vi "Do.vi"(8 "error in (no error)":errorcluster, 10 "Actor in":refnum<class "Actor.lvclass">, 11 "Measure Msg":refnum<class "Measure Msg.lvclass">) -> (0 "error out":errorcluster, 2 "Actor out":refnum<class "Actor.lvclass">)   [LabVIEW 2015, in "Measurement Actor.lvlib" / "Measure Msg.lvclass"]
uses:
  Measure Msg.lvclass
  <vilib>/ActorFramework/Actor/Actor.lvclass
  Measurement.lvclass
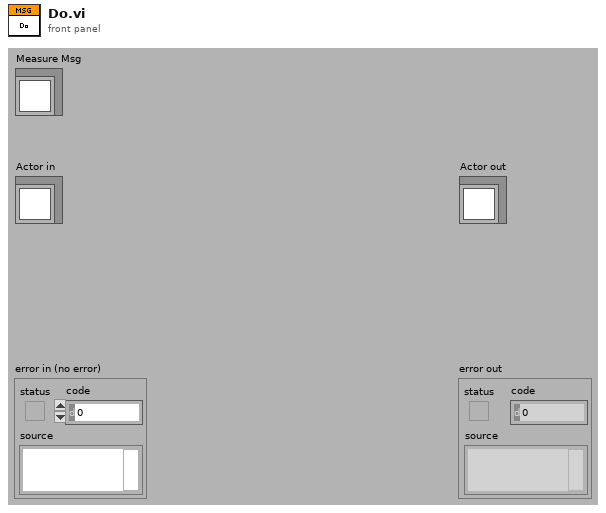
[diagram p1: front panel]
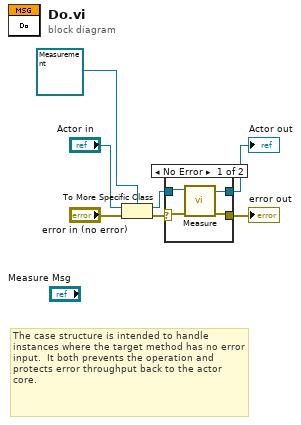
[diagram p0: block diagram]
diagram:
  # "The case structure is intended to handle instances where the target method has no error input.  It both prevents the operation and protects error throughput back to the actor core."
  n1 = To More Specific Class(target class=refnum<class "Measurement.lvclass"> refnum ("Measurement.lvclass"), reference="Actor in", error in="error in (no error)") -> (specific class reference=w7:refnum<class "Measurement.lvclass">, error out=w4:errorcluster)
  n2 = case shown="No Error" w4 {
    selector: w4 -> [w10 w13]
    tunnel: w7 -> [w11 w12]
    tunnel: [w9 w13] -> w3
    tunnel: [w8 w12] -> w2
    frame No Error {
      n3 = call-dynamic "Measure.vi"("error in (no error)"=w10, "Measurement in"=w11) -> ("error out"=w9:errorcluster, "Measurement out"=w8:refnum<class "Measurement.lvclass">)  [unwired: 8 in]
    }
    frame Error {
    }
  }
  "error out" <- w3
  "Actor out" <- w2
